vi "set_output_off.vi"(8 "error in":errorcluster, 11 "VISA resource name":refnum<visa-resource-name>="COM1") -> (0 "error out":errorcluster, 3 "Response":string)   [LabVIEW 2020]
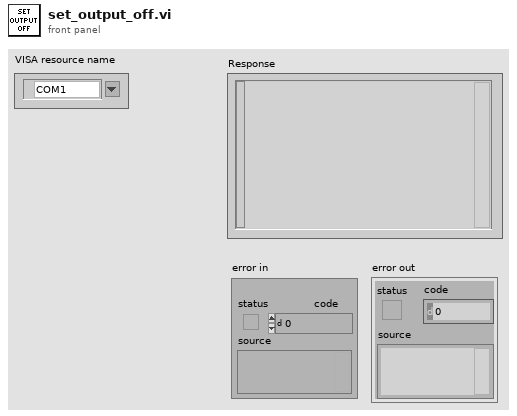
[diagram p1: front panel]
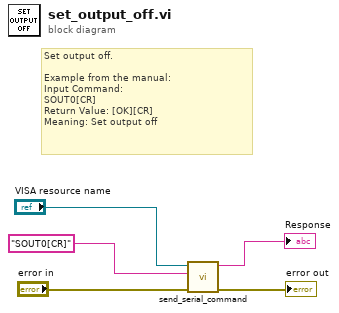
[diagram p0: block diagram]
diagram:
  # "Set output off.\n\nExample from the manual:\nInput Command:\nSOUT0[CR]\nReturn Value: [OK][CR]\nMeaning: Set output off"
  n1 = call "send_serial_command.vi"("error in (no error)"="error in", "Command"="SOUT0[CR]", "VISA resource name"="VISA resource name") -> ("error out"=→"error out":errorcluster, "Response"=→"Response":string)  [unwired: 7 in]
